vi "ТЗЧ_проба.vi"() -> ()   [LabVIEW 2013]
uses:
  <instrlib>/niDMM/nidmm.llb/niDMM Configure Measurement Digits.vi
  <instrlib>/niDMM/nidmm.llb/niDMM Resolution in Digits.ctl
  <instrlib>/niDMM/nidmm.llb/niDMM Function.ctl
panel:
  in  "Param_Log":path=path "D:/#rkm/Фонон-4/ТермоЛазер/Фонон-4_ПОМ_ПрОМ/Прога/ThermoLaser/Logs/Отчетные/Промер до всего/ПОМ"
  in  "№#":i16=20002
  out "4071(1)_adress":refnum<k15>="PXI1Slot4_2 (4)" caption="4071(1)_out"
  in  "4071(1)":refnum<k15>="PXI1Slot4_2"
  out "4070_address":refnum<k15>="PXI1Slot5_2 (4)" caption="4070_out"
  in  "4070":refnum<k15>="PXI1Slot5_2"
  out "Source_2_Vcc_out":refnum<k15> caption="instrument handle out"
  out "Source_1_Vcc_out":refnum<k15> caption="instrument handle out"
  in  "Source_2":refnum<k15>
  in  "Source_1":refnum<k15>="PXI1Slot6"
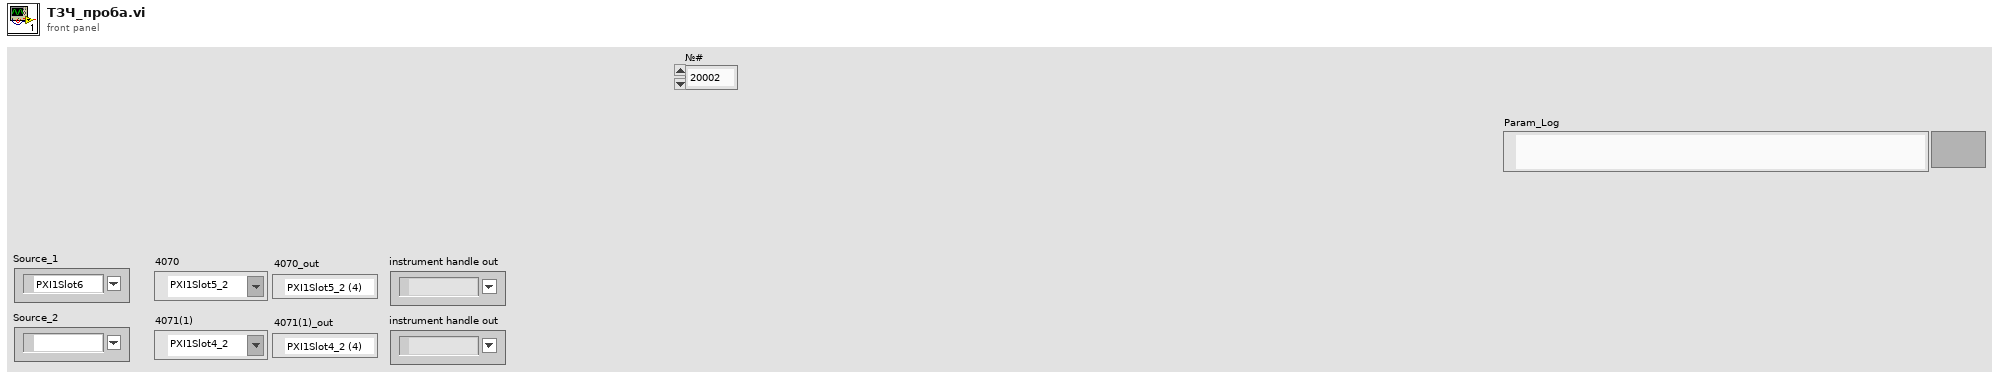
[diagram p1: front panel]
types:
  T1 = enum16{"Инициализация", "Ожидание", "Контроль тока", "Выход"}
  T2 = typedef "niDMM Function.ctl" = enum16{"DC Volts", "AC Volts", "DC Current", "AC Current", "2-wire Resistance", "4-wire Resistance", "Diode", "Frequency", "Period", "AC Volts DC Coupled", "Capacitance", "Inductance", "Temperature"}
  T3 = typedef "niDMM Resolution in Digits.ctl" = dbl
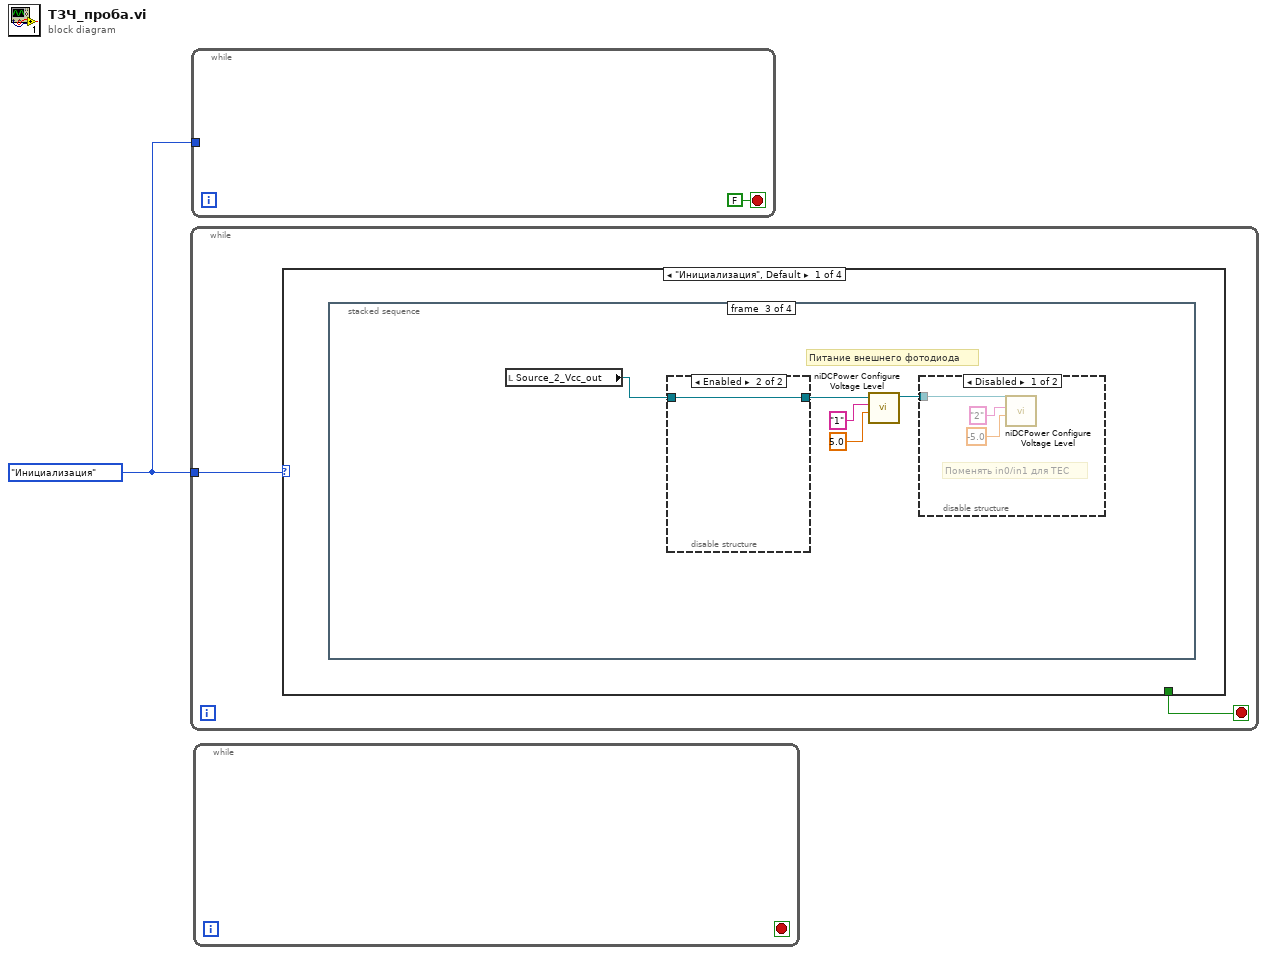
[diagram p0: block diagram]
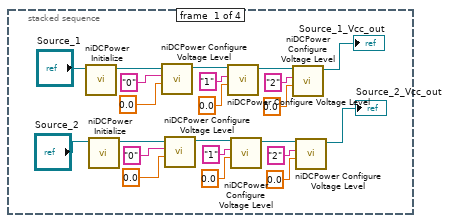
[diagram p2: hidden frame]
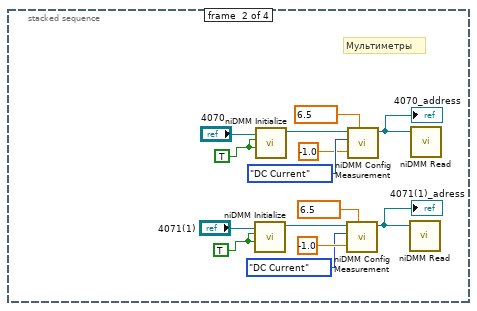
[diagram p3: hidden frame]
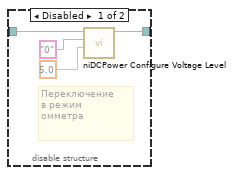
[diagram p4: hidden frame]
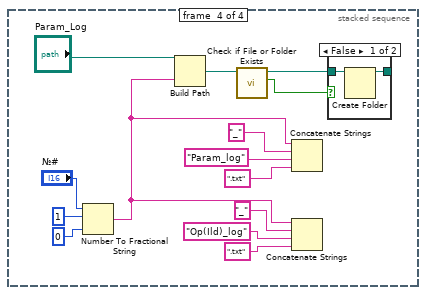
[diagram p6: hidden frame]
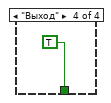
[diagram p10: hidden frame]
diagram:
  w1 = T1."Инициализация"
  n1 = while {
    tunnel: w1 -> [w3]
    stop <- w2 stop-if-true
    n2 = case shown="\"Инициализация\", Default" w3 {
      tunnel: [_ _ _ TRUE] -> w2
      frame "Инициализация", Default {
        n3 = stacked-sequence {
          frame #0 {
            n4 = call <instrlib>:"niDCPower Initialize.vi"("resource name"="Source_1") -> ("instrument handle out"=w23:refnum<k15>)  [unwired: 3 in, 7 out]
            n5 = call <instrlib>:"niDCPower Initialize.vi"("resource name"="Source_2") -> ("instrument handle out"=w9:refnum<k15>)  [unwired: 3 in, 7 out]
            n6 = call <instrlib>:"niDCPower Configure Voltage Level.vi"("voltage level"=0.0, "channel name"="0", "instrument handle"=w23) -> ("instrument handle out"=w24:refnum<k15>)  [unwired: 7 in, 1 out]
            n7 = call <instrlib>:"niDCPower Configure Voltage Level.vi"("voltage level"=0.0, "channel name"="0", "instrument handle"=w9) -> ("instrument handle out"=w8:refnum<k15>)  [unwired: 7 in, 1 out]
            n8 = call <instrlib>:"niDCPower Configure Voltage Level.vi"("voltage level"=0.0, "channel name"="1", "instrument handle"=w24) -> ("instrument handle out"=w19:refnum<k15>)  [unwired: 7 in, 1 out]
            n9 = call <instrlib>:"niDCPower Configure Voltage Level.vi"("voltage level"=0.0, "channel name"="1", "instrument handle"=w8) -> ("instrument handle out"=w12:refnum<k15>)  [unwired: 7 in, 1 out]
            n10 = call <instrlib>:"niDCPower Configure Voltage Level.vi"("voltage level"=0.0, "channel name"="2", "instrument handle"=w19) -> ("instrument handle out"=→"Source_1_Vcc_out":refnum<k15>)  [unwired: 7 in, 1 out]
            n11 = call <instrlib>:"niDCPower Configure Voltage Level.vi"("voltage level"=0.0, "channel name"="2", "instrument handle"=w12) -> ("instrument handle out"=→"Source_2_Vcc_out":refnum<k15>)  [unwired: 7 in, 1 out]
          }
          frame #1 {
            w26 = T3 6.5 items=["3 1/2"=3.5, "4 1/2"=4.5, "5 1/2"=5.5, "6 1/2"=6.5, "7 1/2"=7.5] ("Resolution in Digits")
            w28 = TRUE ("Reset")
            w39 = T3 6.5 items=["3 1/2"=3.5, "4 1/2"=4.5, "5 1/2"=5.5, "6 1/2"=6.5, "7 1/2"=7.5] ("Resolution in Digits")
            w37 = TRUE ("Reset")
            # "Мультиметры"
            n12 = call <instrlib>:"niDMM Initialize.vi"("Reset"=w28, "ID Query"=w28, "Instrument Descriptor"="4071(1)") -> ("instrument handle out"=w30:refnum<k15>)  [unwired: 7 in, 1 out]
            n13 = call <instrlib>:"niDMM Initialize.vi"("Reset"=w37, "ID Query"=w37, "Instrument Descriptor"="4070") -> ("instrument handle out"=w35:refnum<k15>)  [unwired: 7 in, 1 out]
            n14 = call-poly <instrlib>:"niDMM Config Measurement.vi"("Range"=-1.0 ("Configuration:Measurement Options:Max Frequency"), "Resolution in Digits"=w26, "Function"=niDMM_Function."DC Current" ("multimeter mode"), "instrument handle"=w30) -> ("instrument handle out"=w32:refnum<k15>)  [unwired: 6 in, 1 out]
            "4071(1)_adress" <- w32
            n15 = call-poly <instrlib>:"niDMM Config Measurement.vi"("Range"=-1.0 ("Configuration:Measurement Options:Max Frequency"), "Resolution in Digits"=w39, "Function"=niDMM_Function."DC Current" ("multimeter mode"), "instrument handle"=w35) -> ("instrument handle out"=w33:refnum<k15>)  [unwired: 6 in, 1 out]
            "4070_address" <- w33
            n16 = call <instrlib>:"niDMM Read.vi"("instrument handle"=w32) -> ()  [unwired: 8 in, 3 out]
            n17 = call <instrlib>:"niDMM Read.vi"("instrument handle"=w33) -> ()  [unwired: 8 in, 3 out]
          }
          frame #2 {
            # "Питание внешнего фотодиода"
            n18 = local read "Source_2_Vcc_out"() -> (w44:refnum<k15>)
            n19 = disable-structure shown="Enabled" {
              disable-tunnel: w44 -> [w48 w49]
              disable-tunnel: [w47 w49] -> w43
              frame Disabled {
                # "Переключение\nв режим\nомметра"
                n20 = call <instrlib>:"niDCPower Configure Voltage Level.vi"("voltage level"=5.0, "channel name"="0", "instrument handle"=w48) -> ("instrument handle out"=w47:refnum<k15>)  [unwired: 7 in, 1 out]
              }
              frame Enabled {
              }
            }
            n21 = call <instrlib>:"niDCPower Configure Voltage Level.vi"("voltage level"=5.0, "channel name"="1", "instrument handle"=w43) -> ("instrument handle out"=w42:refnum<k15>)  [unwired: 7 in, 1 out]
            n22 = disable-structure shown="Disabled" {
              disable-tunnel: w42 -> [w52 _]
              frame Disabled {
                # "Поменять in0/in1 для ТЕС"
                n23 = call <instrlib>:"niDCPower Configure Voltage Level.vi"("voltage level"=-5.0, "channel name"="2", "instrument handle"=w52) -> ()  [unwired: 7 in, 2 out]
              }
              frame Enabled {
              }
            }
          }
          frame #3 {
            n24 = Number To Fractional String(number="№#", width (-)=i16 1, precision (6)=i16 0) -> (F-format string=w68:string)  [unwired: 1 in]
            n25 = Build Path(base path="Param_Log", name or relative path=w68) -> (appended path=w57:path)
            n26 = call <vilib>:"Check if File or Folder Exists.vi"("path"=w57) -> ("file or folder exists?"=w59:bool, "dup path"=w58:path)  [unwired: 8 in, 1 out]
            n27 = Concatenate Strings(w68, "_" ("element"), "Param_log" ("string"), ".txt" ("element")) -> (w62:string)
            n28 = Concatenate Strings(w68, "_" ("element"), "Op(Ild)_log" ("string"), ".txt" ("element")) -> (w53:string)
            n29 = case shown="False" w59 {
              tunnel: w58 -> [w71 w72]
              tunnel: [w70 w72] -> w69
              frame False {
                n30 = Create Folder(path (use dialog)=w71) -> (created path=w70:path)  [unwired: 2 in, 2 out]
              }
              frame True {
              }
            }
          }
        }
      }
      frame "Ожидание" {
      }
      frame "Контроль тока" {
      }
      frame "Выход" {
      }
    }
  }
  n31 = while {
    tunnel: w1 -> [_]
    stop <- FALSE stop-if-true
  }
  n32 = while {
    stop <- _ stop-if-true
  }
